vi "Reconstruct ROI group image.vi"(8 "error in":errorcluster, 11 "Name of ROI group to search for":string) -> (0 "error out":errorcluster, 2 "Red & Green ROI group image cluster":T2, 3 "Image to display":T1)   [LabVIEW 2020]
uses:
  <vilib>/vision/Image Controls.llb/IMAQ Image.ctl
  Typedefs/Get-Set-Clear Control.ctl
  Typedefs/ROI parameters data type.ctl
  Global variables/gl_Functional Imaging-Global variables.vi
  <vilib>/vision/NI_Vision_Development_Module.lvlib
panel:
  out "Multiple Z-planes added":bool
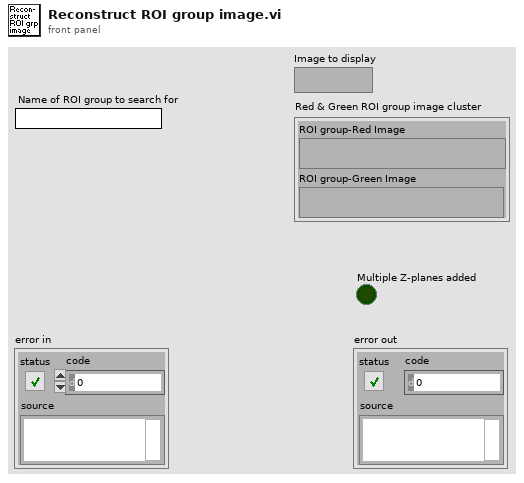
[diagram p1: front panel]
types:
  T1 = typedef "IMAQ Image.ctl" = refnum<image>
  T2 = cluster{"ROI group-Red Image":T1, "ROI group-Green Image":T1}
  T3 = typedef "Get-Set-Clear Control.ctl" = enum16{"Get", "Set", "Clear"}
  T4 = typedef "ROI parameters data type.ctl" = cluster{"ROI index":dbl, "ROI ID":dbl, "ROI Time (ns)":dbl, "Pixels in ROI":dbl, "X start":dbl, "Y start":dbl, "Z start":dbl, "X stop":dbl, "Y stop":dbl, "Z stop":dbl, "Angle (deg)":dbl, "Composite ID":dbl, "Number of lines":dbl, "Frame Size":dbl, "Zoom":dbl, "Laser Power (%)":dbl, "ROI group ID":dbl, "Resolution":dbl, "Dwell Time per pixel":dbl, "Pixels per miniscan":dbl, "Original FOV (um)":dbl, "Apparent Frame Size":dbl, "Z Plane Idx":i32[], "Z Plane codes":i32[]}
  T5 = enum32{"Average", "Min", "Max", "Clear  if < ", "Clear  if < or =", "Clear  if =", "Clear  if > or =", "Clear  if >"}
  T6 = typedef "Image Type" = u32
  T7 = typedef "ROI group info cluster.ctl" = cluster{"Group name":string, "# ROI in group":i32, "ROI numbers in group":i32[], "Group region specifier cluster":T8}
  T8 = typedef "ROI Descriptor" = cluster{"Global Rectangle":i32[], "Contours":cluster{"ID":enum32{"External", "Internal"}, "Type":u32, "Coordinates":i32[]}[]}
  T9 = typedef "Functional Parameters Cluster.ctl" = cluster{"ROI data":dbl[][], "ROI format version":i32, "Norm ROI data":dbl[][], "Norm. ROI format version":i32, "Z norm":dbl[], "Z norm format version":i32}
  T10 = typedef "Fixed strings.ctl" = cluster{"ROI file name":string, "Normalised ROI file name":string, "Zplane Pockels values file name":string, "Functional data folder name":string, "Experiment Header file name":string, "Z-stack images folder name":string, "Groups setup rel. path":string, "Groups text file rel. path":string, "TDMS files folder name (F.img)":string, "TDMS files folder name (V.acq)":string, "TDMS files folder name (Pl.acq)":string, "Cycle rel times sequence file":string, "Dynamically called VIs folder name":string, "Time Series folder base name":string}
  T11 = typedef "Functional Imging UI Refs.ctl" = cluster{"Menu ref":refnum<k9>, "Image control":refnum<vi>, "VI ref":refnum<vi>, "XGrapher":refnum<vi>, "Smoothing":refnum<vi>, "POI Averaging":refnum<vi>, "Normalize":refnum<vi>, "POI data points in each trial":refnum<vi>, "Channel":refnum<vi>, "Experiment data folder path":refnum<vi>, "[ROI vis]":refnum<vi>, "[Groups] visbl":T12, "Group Name":refnum<vi>, "POI index":refnum<vi>, "Trial No.":refnum<vi>, "Intensity Zoom":refnum<vi>, "Trial Cursor Enabled":refnum<vi>, "Number of Trials (ind 1)":refnum<vi>, "Number of Trials (ind 2)":refnum<vi>, "MiniScans Available":refnum<vi>, "POI Available":refnum<vi>, "Defer graph updates":refnum<vi>, "Waveform selector":refnum<vi>, "#of selected POI":refnum<vi>, "#of selected MiniScans":refnum<vi>, "#of selected groups":refnum<vi>, "Max Z-Projection":refnum<vi>, "Z-Plane Selector":refnum<vi>, "Index of miniscan point to visualise":refnum<vi>, "ROI vis. mode":refnum<vi>, "Total # of points":refnum<vi>, "Index of group clicked on":refnum<vi>, "Pane 1":refnum<vi>, "Pane 2":refnum<vi>, "Pane 3":refnum<vi>, "Pane 4":refnum<vi>, "Pane 5":refnum<vi>, "Pane 6":refnum<vi>, "Deselect all ROI":refnum<vi>, "Deselect all groups":refnum<vi>}
  T12 = typedef "Groups array referecne.ctl" = refnum<vi>
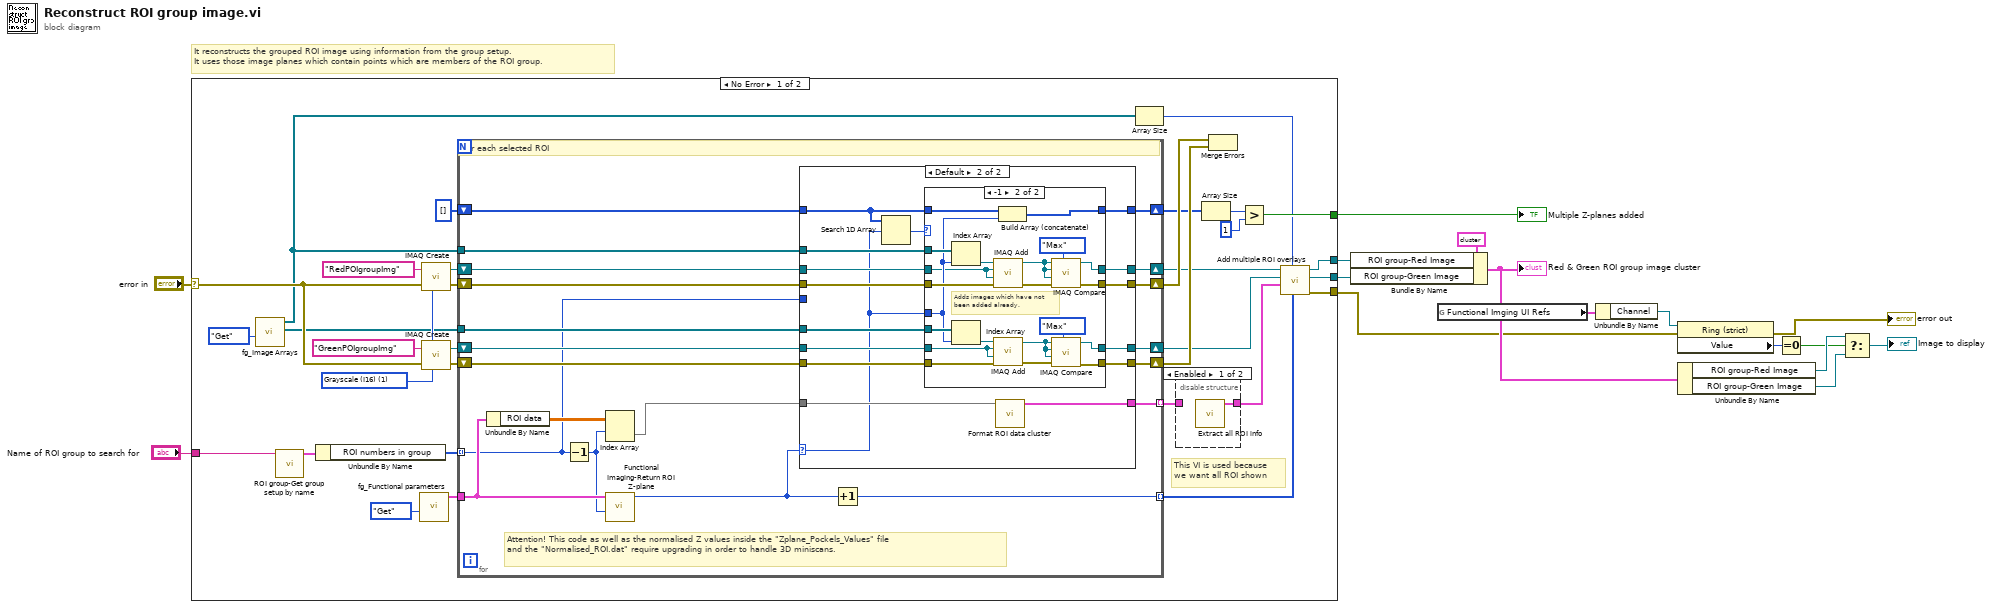
[diagram p0: block diagram]
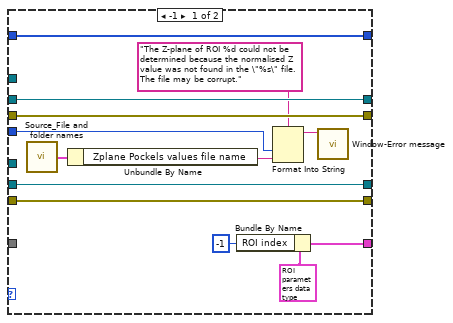
[diagram p3: hidden frame]
diagram:
  # "It reconstructs the grouped ROI image using information from the group setup.\nIt uses those image planes which contain points which are members of the ROI group."
  n1 = case shown="No Error" "error in" {
    selector: "error in" -> [w41 w126]
    tunnel: [w33 _] -> w12
    tunnel: [w34 _] -> w13
    tunnel: [w31 w126] -> w5
    tunnel: [w40 _] -> w15
    tunnel: "Name of ROI group to search for" -> [w17 _]
    frame No Error {
      w48 = T6 1 items=["Grayscale (U8)", "Grayscale (I16)", "Grayscale (SGL)", "Complex (CSG)", "RGB (U32)", "HSL (U32)", "RGB (U64)"] ("Image Type")
      # "This VI is used because\nwe want all ROI shown"
      n2 = call "fg_Image Arrays.vi"("Function"=Get-Set-Clear_Control."Get") -> ("Green Images Array"=w35:T1[], "Red Images Array"=w36:T1[])  [unwired: 9 in]
      n3 = call "ROI group-Get group setup by name.vi"("Name of ROI group to search for"=w17) -> ("POI group info cluster"=w18:T7)  [unwired: 8 in, 2 out]
      n4 = Unbundle By Name(w18) -> ("ROI numbers in group"=w23:i32[])
      n5 = call "fg_Functional parameters.vi"("Function"=Get-Set-Clear_Control."Get") -> ("Functional Parameters"=w37:T9)  [unwired: 7 in, 3 out]
      n6 = call "IMAQ Create"("Image Name"="RedPOIgroupImg" ("string"), "Image Type"=w48, "error in (no error)"=w41) -> ("New Image"=w42:T1, "error out"=w43:errorcluster)  [unwired: 2 in]
      n7 = call "IMAQ Create"("Image Name"="GreenPOIgroupImg" ("string"), "Image Type"=w48, "error in (no error)"=w41) -> ("New Image"=w45:T1, "error out"=w44:errorcluster)  [unwired: 2 in]
      n8 = for {
        shift-right: [w66] -> w21
        shift-left: w45 -> [w61]
        shift-right: [w67] -> w22
        shift-left: w42 -> [w58]
        tunnel: w36 -> [w63]
        tunnel: w35 -> [w68]
        tunnel: w23 -> [w51] mode=indexing
        tunnel: [w60] -> w19 mode=indexing
        shift-right: [w64] -> w29
        shift-left: w43 -> [w69]
        shift-right: [w65] -> w28
        shift-left: w44 -> [w70]
        tunnel: w37 -> [w54]
        tunnel: [w57] -> w32 mode=indexing
        shift-right: [w56] -> w26
        shift-left: i32[] [] -> [w55]
        # "Attention! This code as well as the normalised Z values inside the \"Zplane_Pockels_Values\" file\nand the \"Normalised_ROI.dat\" require upgrading in order to handle 3D miniscans."
        # "For each selected ROI"
        n9 = Unbundle By Name(w54) -> ("ROI data"=w59:dbl[][])
        n10 = Decrement(x=w51) -> (x-1=w53:i32)
        n11 = Index Array(array=w59, index (row)=w53) -> (element=w62:dbl[])  [unwired: 1 in]
        n12 = call "Functional Imaging-Return ROI Z-plane.vi"("ROI index (zero based)"=w53, "Functional Parameters"=w54) -> ("Zero-based index of the Z-plane the indexed ROI belongs to"=w52:i32)  [unwired: 9 in]
        n13 = case shown="Default" w52 {
          selector: w52 -> [_ w84]
          tunnel: w70 -> [w80 w92]
          tunnel: w69 -> [w81 w93]
          tunnel: w68 -> [_ w99]
          tunnel: [w83 w98] -> w67
          tunnel: [w82 w97] -> w66
          tunnel: [w80 w96] -> w65
          tunnel: [w81 w95] -> w64
          tunnel: w63 -> [_ w94]
          tunnel: w62 -> [_ w88]
          tunnel: w61 -> [w82 w91]
          tunnel: [w77 w89] -> w60
          tunnel: w58 -> [w83 w90]
          tunnel: w51 -> [w76 _]
          tunnel: [w74 w87] -> w56
          tunnel: w55 -> [w74 w86]
          frame -1 {
            n14 = call "Source_File and folder names.vi"() -> ("Fixed strings"=w71:T10)  [unwired: 1 in]
            n15 = Unbundle By Name(w71) -> ("Zplane Pockels values file name"=w73:string)
            n16 = Bundle By Name(cluster=T4 {"ROI index"=0.0, "ROI ID"=0.0, "ROI Time (ns)"=0.0, "Pixels in ROI"=0.0, "X start"=0.0, "Y start"=0.0, "Z start"=0.0, "X stop"=0.0, "Y stop"=0.0, "Z stop"=0.0, "Angle (deg)"=0.0, "Composite ID"=0.0, "Number of lines"=0.0, "Frame Size"=0.0, "Zoom"=0.0, "Laser Power (%)"=0.0, "ROI group ID"=0.0, "Resolution"=0.0, "Dwell Time per pixel"=0.0, "Pixels per miniscan"=0.0, "Original FOV (um)"=0.0, "Apparent Frame Size"=0.0, "Z Plane Idx"=[], "Z Plane codes"=[]} ("X-Y-Z coordinates"), "ROI index"=i64 -1) -> (w77:T4)
            n17 = Format Into String(format string="The Z-plane of ROI %d could not be determined because the normalised Z value was not found in the \"%s\" file. The file may be corrupt." ("message"), w76, w73) -> (resulting string=w72:string)  [unwired: 2 in, 1 out]
            n18 = call "Window-Error message.vi"("Message"=w72) -> ()  [unwired: 10 in, 1 out]
          }
          frame Default {
            n19 = Search 1D Array(1D array=w86, element=w84) -> (index of element=w85:i32)  [unwired: 1 in]
            n20 = case shown="-1" w85 {
              tunnel: w99 -> [_ w123]
              tunnel: [w104 w122] -> w98
              tunnel: [w103 w121] -> w97
              tunnel: [w101 w120] -> w96
              tunnel: [w102 w119] -> w95
              tunnel: w94 -> [_ w118]
              tunnel: w84 -> [_ w107]
              tunnel: w93 -> [w102 w117]
              tunnel: w92 -> [w101 w116]
              tunnel: w91 -> [w103 w114]
              tunnel: w90 -> [w104 w105]
              tunnel: [w100 w108] -> w87
              tunnel: w86 -> [w100 w106]
              frame Default {
                # "Image already added."
              }
              frame -1 {
                # "Adds images which have not\nbeen added already."
                n21 = Index Array(array=w118, index=w107) -> (element=w110:T1)
                n22 = Index Array(array=w123, index=w107) -> (element=w115:T1)
                n23 = call "IMAQ Add"("Image Src A"=w110, "Image Dst"=w105, "Image Src B"=w105, "error in (no error)"=w117) -> ("Image Dst Out"=w109:T1, "error out"=w112:errorcluster)  [unwired: 3 in]
                n24 = call "IMAQ Add"("Image Src A"=w115, "Image Dst"=w114, "Image Src B"=w114, "error in (no error)"=w116) -> ("Image Dst Out"=w113:T1, "error out"=w111:errorcluster)  [unwired: 3 in]
                n25 = Build Array (concatenate)(w106, w107) -> (w108:i32[])
                n26 = call "IMAQ Compare"("Operator"=T5."Max", "error in (no error)"=w112, "Image Src B"=w109, "Image Dst"=w109, "Image Src A"=w109) -> ("error out"=w119:errorcluster, "Image Dst Out"=w122:T1)  [unwired: 5 in]
                n27 = call "IMAQ Compare"("Operator"=T5."Max", "error in (no error)"=w111, "Image Src B"=w113, "Image Dst"=w113, "Image Src A"=w113) -> ("error out"=w120:errorcluster, "Image Dst Out"=w121:T1)  [unwired: 5 in]
              }
            }
            n28 = call "Format ROI data cluster.vi"("Single ROI info"=w88) -> ("X-Y-Z coordinates"=w89:T4)  [unwired: 10 in]
          }
        }
        n29 = Increment(x=w52) -> (x+1=w57:i32)
      }
      n30 = Array Size(array=w36) -> (size(s)=w30:i32)
      n31 = disable-structure shown="Enabled" {
        disable-tunnel: [w49 w50] -> w20
        disable-tunnel: w19 -> [_ w50]
        frame Enabled {
          n32 = call "Extract all ROI info.vi"() -> ("[ROI info]"=w49:T4[])  [unwired: 10 in, 1 out]
        }
        frame Disabled {
        }
      }
      n33 = Array Size(array=w26) -> (size(s)=w25:i32)
      n34 = Merge Errors(w29, w28) -> ()  [unwired: 1 out]
      n35 = Greater?(x=w25, y=1) -> (0:w40:bool)
      n36 = call "Add multiple ROI overlays.vi"("[ROI index] (unity based)"=w32, "# of Z-planes"=w30, "[ROI info]"=w20, "Image 2 in"=w21, "Image 1 in"=w22) -> ("error out"=w31:errorcluster, "Image 2 out"=w33:T1, "Image 1 out"=w34:T1)  [unwired: 4 in]
    }
    frame Error {
    }
  }
  "Multiple Z-planes added" <- w15
  n37 = Bundle By Name(cluster=T2 {"ROI group-Red Image"=refnum, "ROI group-Green Image"=refnum} ("Red & Green ROI group image cluster"), "ROI group-Red Image"=w13, "ROI group-Green Image"=w12) -> (w6:T2)
  "Red & Green ROI group image cluster" <- w6
  n38 = global read "gl_Functional Imaging-Global variables.vi" "Functional Imging UI Refs"() -> (w7:T11)
  n39 = Unbundle By Name(w7) -> ("Channel"=w3:refnum<vi>)
  n40 = property on="Property Node" class="Ring (strict)"(reference=w3, error in=w5) -> (error out=→"error out":errorcluster, "Value"=w11:u16)  [unwired: 1 out]
  n41 = Unbundle By Name(w6) -> ("ROI group-Red Image"=w10:T1, "ROI group-Green Image"=w9:T1)
  n42 = Equal To 0?(x=w11) -> (x = 0?=w8:bool)
  n43 = Select(t=w10, s=w8, f=w9) -> (s? t:f=→"Image to display":T1)
